vi "Calculate Maximum Deviation.vi"(2 "Sample":dbl[](array[numeric]), 3 "fine":i32) -> (0 "number of samples":i32, 1 "Outliers":dbl)   [LabVIEW 2013]
panel:
  out "Sums":dbl[](array[numeric])
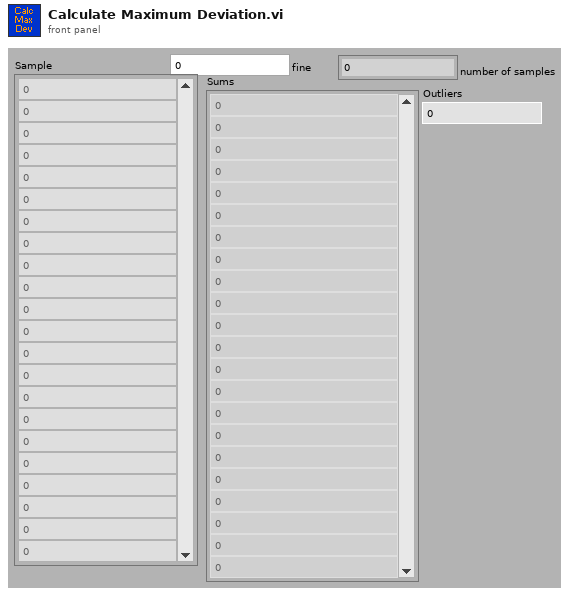
[diagram p1: front panel]
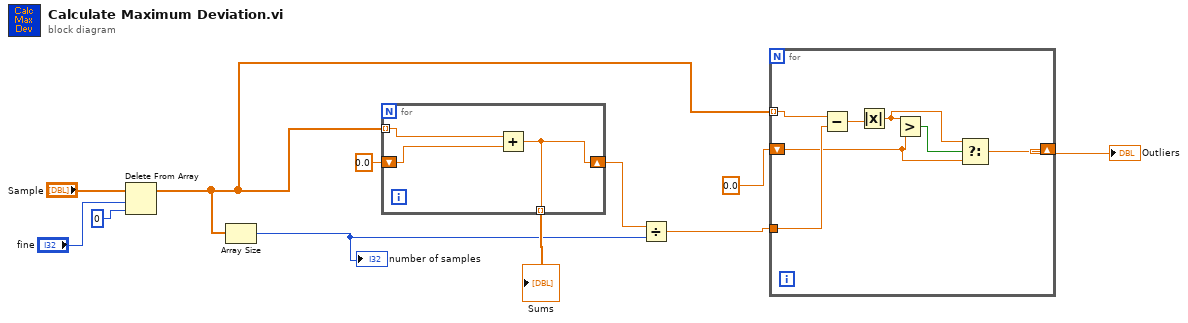
[diagram p0: block diagram]
diagram:
  n1 = Delete From Array(array="Sample", length="fine", index=0 ("disabled index (col)")) -> (array with subset deleted=w4:dbl[])  [unwired: 1 out]
  n2 = Array Size(array=w4) -> (size(s)=w3:i32)
  "number of samples" <- w3
  n3 = for {
    tunnel: w4 -> [w14] mode=indexing
    shift-right: [w12] -> w11
    shift-left: 0.0 -> [w13]
    tunnel: [w12] -> w6 mode=indexing
    n4 = Add(x=w14, y=w13) -> (x+y=w12:dbl)
  }
  "Sums" <- w6
  n5 = Divide(x=w11, y=w3) -> (x/y=w9:dbl)
  n6 = for {
    tunnel: w4 -> [w21] mode=indexing
    tunnel: w9 -> [w20]
    shift-right: [w16] -> w8
    shift-left: 0.0 ("element") -> [w17]
    n7 = Subtract(x=w21, y=w20) -> (x-y=w19:dbl)
    n8 = Absolute Value(x=w19) -> (abs(x)=w18:dbl)
    n9 = Greater?(x=w18, y=w17) -> (0:w15:bool)
    n10 = Select(t=w18, s=w15, f=w17) -> (s? t:f=w16:dbl)
  }
  "Outliers" <- w8
